vi "Select_Coreset_Idxs(CuLab).vi"(8 "error in (no error)":errorcluster, 9 "start idx":i32=-1, 10 "Sampling Ratio":sgl format="%#_13g", 11 "Features (embeddings)":refnum<class "T2D_SGL.lvclass">) -> (0 "error out":errorcluster, 2 "max distances":refnum<class "T1D_SGL.lvclass">, 3 "selected coreset idxs":i32[](array[numeric]))   [LabVIEW 2020]
uses:
  <vilib>/Ngene/CuLab - GPU Accelerated Toolkit/Toolkit/Low_Level/Tensor_Classes/T_Children/T2D/T2D_Children/T2D_SGL/T2D_SGL.lvclass
  C:/Program Files/National Instruments/LabVIEW 2020/vi.lib/Ngene/CuLab - GPU Accelerated Toolkit/Toolkit/Low_Level/Tensor_Classes/T_Children/T2D/T2D.lvclass
  <vilib>/Ngene/CuLab - GPU Accelerated Toolkit/Toolkit/Low_Level/Tensor_Classes/T_Children/T1D/T1D_Children/T1D_SGL/T1D_SGL.lvclass
  C:/Program Files/National Instruments/LabVIEW 2020/vi.lib/Ngene/CuLab - GPU Accelerated Toolkit/Toolkit/Low_Level/Tensor_Classes/T_Children/T1D/T1D.lvclass
  C:/Program Files/National Instruments/LabVIEW 2020/vi.lib/Ngene/CuLab - GPU Accelerated Toolkit/Toolkit/Low_Level/Tensor_Classes/Tensor.lvclass
  <vilib>/Ngene/CuLab - GPU Accelerated Toolkit/Toolkit/API/Array/Controls/Array_Major.ctl
  <vilib>/Ngene/CuLab - GPU Accelerated Toolkit/Toolkit/API/Array/Array Size/CU_Array_Size_T2D.vi
  <vilib>/Ngene/CuLab - GPU Accelerated Toolkit/Toolkit/API/Signal Processing/Signal Generation/Ramp Pattern/T1D/CU_Ramp_Pattern_T1D_SGL.vi
  <vilib>/Ngene/CuLab - GPU Accelerated Toolkit/Toolkit/API/Numeric/Conversion  (API)/I32/CU_To_I32_T1D.vi
  <vilib>/Ngene/CuLab - GPU Accelerated Toolkit/Toolkit/Low_Level/Tensor_Classes/T_Children/T1D/T1D_Children/T1D_I32/Pull.vi
  <vilib>/Ngene/CuLab - GPU Accelerated Toolkit/Toolkit/API/Numeric/Square/T2D/CU_Square_T2D_SGL.vi
  <vilib>/Ngene/CuLab - GPU Accelerated Toolkit/Toolkit/API/Array/Array Size/CU_Array_Size_T1D.vi
  <vilib>/Ngene/CuLab - GPU Accelerated Toolkit/Toolkit/API/Array/Index Array Subset/T2D/CU_Index_Array_Subset_T2D_SGL.vi
  <vilib>/Ngene/CuLab - GPU Accelerated Toolkit/Toolkit/API/Comparison/Max Min/T1D/CU_Max_Min_T1D_SGL.vi
  <vilib>/Ngene/CuLab - GPU Accelerated Toolkit/Toolkit/API/Array/Array Max Min/T1D/CU_Array_Max_Min_T1D_SGL.vi
  <vilib>/Ngene/CuLab - GPU Accelerated Toolkit/Toolkit/API/Array/Replace Array Element/T1D/CU_Replace_Array_Element_T1D_SGL.vi
  <vilib>/Ngene/CuLab - GPU Accelerated Toolkit/Toolkit/CuLab.lvlib
  C:/Program Files/National Instruments/LabVIEW 2020/vi.lib/Ngene/CuLab - GPU Accelerated Toolkit/Toolkit/Low_Level/Tensor_Classes/T_Children/T2D/T2D_Children/T2D_SGL/T2D_SGL.lvclass
  C:/Program Files/National Instruments/LabVIEW 2020/vi.lib/Ngene/CuLab - GPU Accelerated Toolkit/Toolkit/Low_Level/Tensor_Classes/T_Children/T1D/T1D_Children/T1D_SGL/T1D_SGL.lvclass
  <vilib>/Ngene/CuLab - GPU Accelerated Toolkit/Toolkit/Low_Level/Tensor_Classes/T_Children/T1D/T1D_Children/T1D_I32/T1D_I32.lvclass
  <vilib>/Ngene/Deep Learning Toolkit/Toolkit/Deep_Learning_Toolkit_by_Ngene.lvlib
panel:
  out "min distances":refnum<class "T1D_SGL.lvclass">
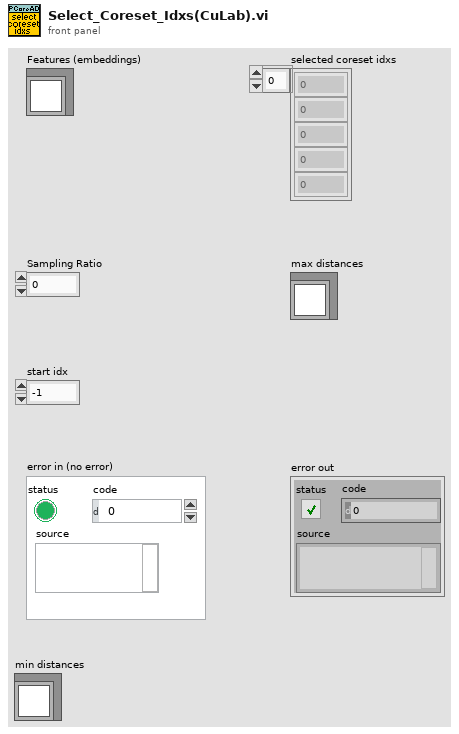
[diagram p1: front panel]
types:
  T1 = typedef "CuLab.lvlib/Array_Major.ctl" = enum16{"Row", "Column"}
  T2 = typedef "CuLab.lvlib/T2D_Dims.ctl" = cluster{"H":i32, "W":i32}
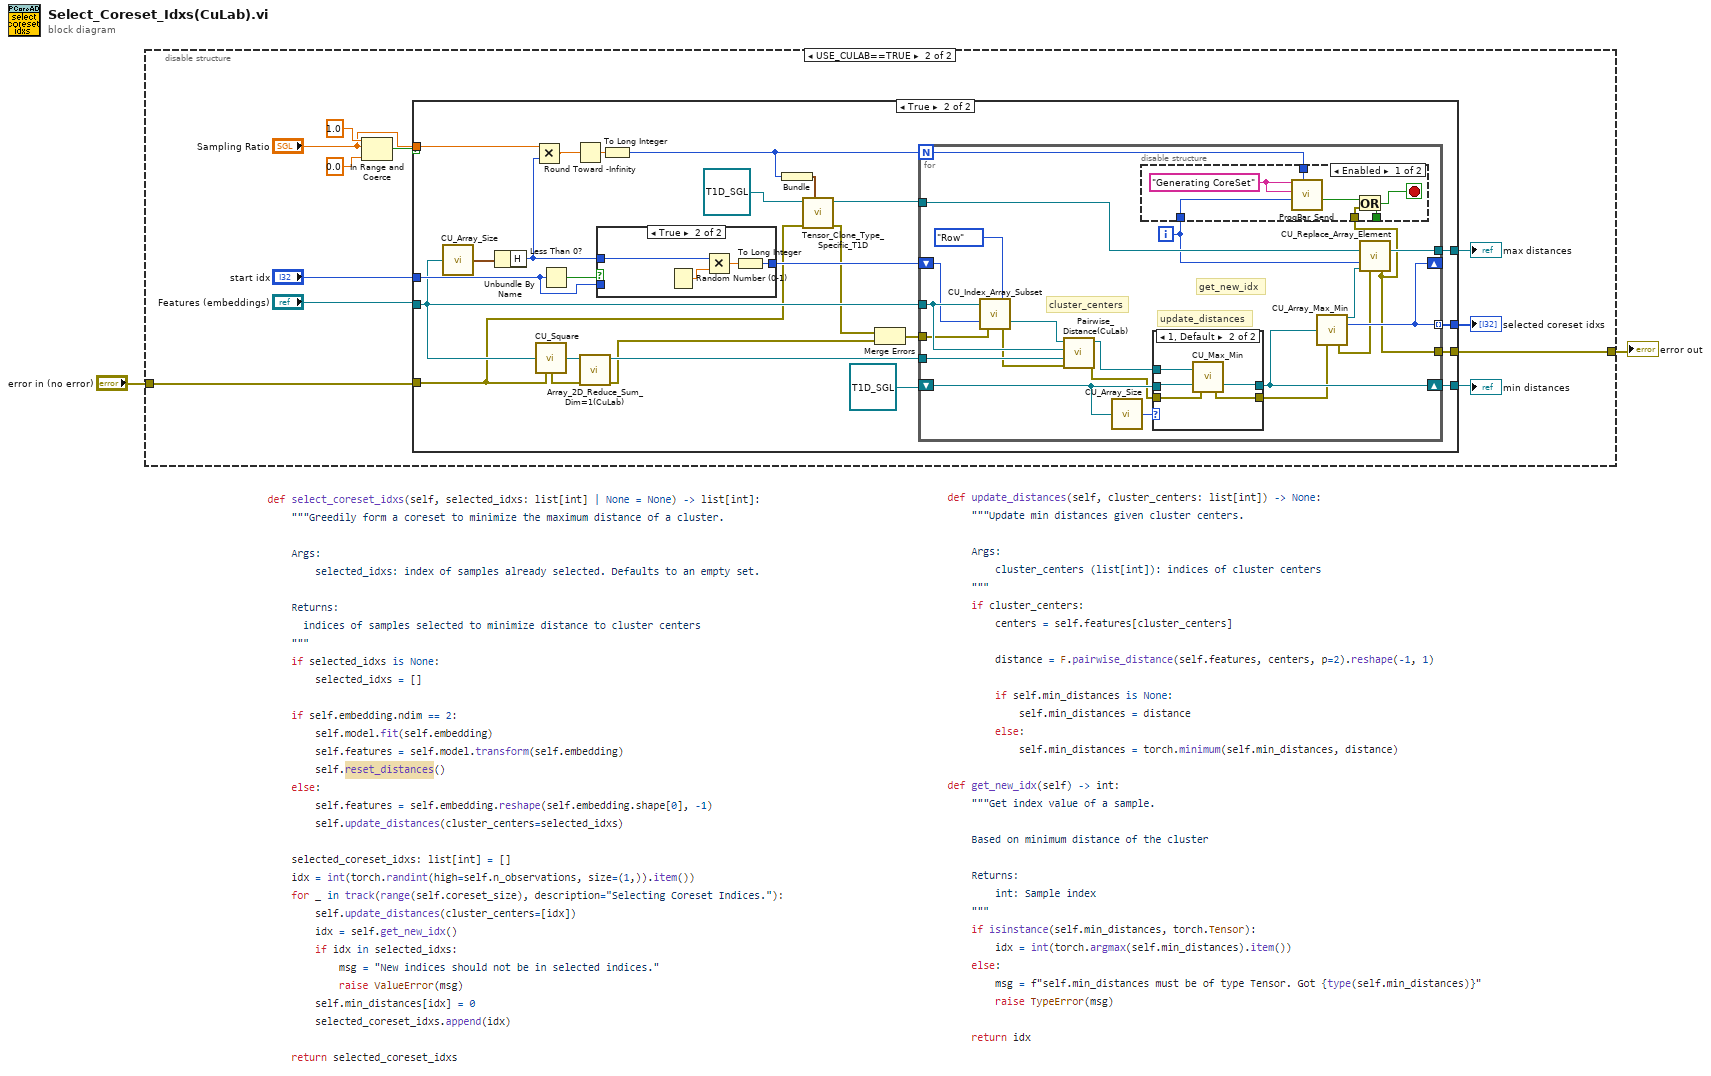
[diagram p0: block diagram]
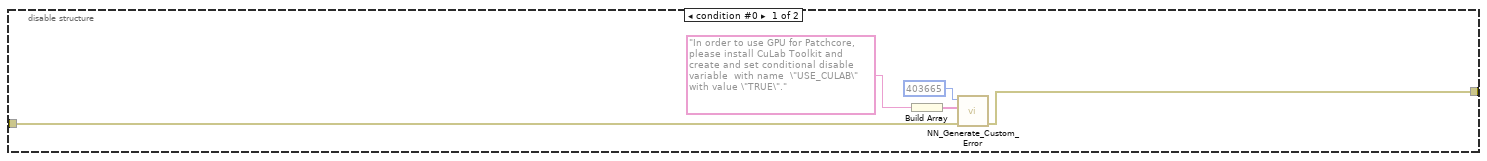
[diagram p2: hidden frame]
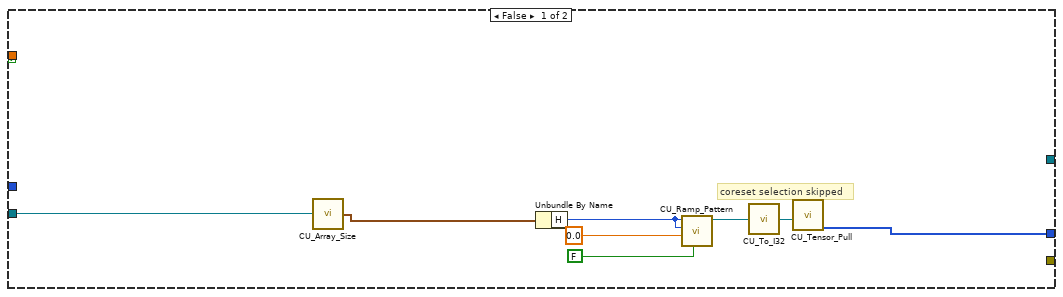
[diagram p3: hidden frame]
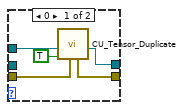
[diagram p6: hidden frame]
diagram:
  n1 = disable-structure shown="USE_CULAB==TRUE" {
    disable-tunnel: [w3 w9] -> w2
    disable-tunnel: "error in (no error)" -> [w4 w8]
    frame condition #0 {
      n2 = Build Array("In order to use GPU for Patchcore, please install CuLab Toolkit and create and set conditional disable variable  with name  \"USE_CULAB\" with value \"TRUE\"." ("Message")) -> (w6:string[])
      n3 = call <vilib>:"NN_Generate_Custom_Error.vi"("error in (no error)"=w4, "Message"=w6, "Error_code"=403665) -> ("error out"=w3:errorcluster)  [unwired: 8 in]
    }
    frame condition #1 (active) {
      n4 = In Range and Coerce(upper limit=sgl 1.0, x="Sampling Ratio", lower limit=sgl 0.0) -> (In Range?=w12:bool)  [unwired: 1 out]
      n5 = case shown="True" w12 {
        tunnel: [w20 w51] -> w18
        tunnel: [_ w50] -> w17
        tunnel: "start idx" -> [_ w47]
        tunnel: "Features (embeddings)" -> [w25 w39]
        tunnel: "Sampling Ratio" -> [_ w42]
        tunnel: [_ w33] -> w10
        tunnel: w8 -> [_ w31]
        tunnel: [_ w28] -> w9
        frame False {
          # "coreset selection skipped"
          n6 = call-poly <vilib>:"CU_Array_Size.vi"("Tensor"=w25) -> ("T2D_Dims"=w26:T2)  [unwired: 14 in]
          n7 = Unbundle By Name(w26) -> ("H"=w19:i32)
          n8 = call-poly <vilib>:"CU_Ramp_Pattern.vi"("exclude end?"=FALSE, "start"=sgl 0.0, "end"=w19, "samples"=w19) -> ("Ramp Pattern"=w22:refnum<class "T1D_SGL.lvclass">)  [unwired: 6 in, 1 out]
          n9 = call-poly <vilib>:"CU_To_I32.vi"("Tensor in"=w22) -> ("Dest out"=w21:refnum<class "T1D_I32.lvclass">)  [unwired: 13 in, 1 out]
          n10 = call-poly <vilib>:"CU_Tensor_Pull.vi"("T1D_I32 in"=w21) -> ("Dest out"=w20:i32[])  [unwired: 8 in, 2 out]
        }
        frame True {
          n11 = call-poly <vilib>:"CU_Array_Size.vi"("Tensor"=w39) -> ("T2D_Dims"=w41:T2)  [unwired: 14 in]
          n12 = Unbundle By Name(w41) -> ("H"=w40:i32)
          n13 = Multiply(x=w42, y=w40) -> (x*y=w43:sgl)
          n14 = call-poly <vilib>:"CU_Square.vi"("x"=w39, "error in (no error)"=w31) -> ("Dest out"=w46:refnum<class "T2D_SGL.lvclass">, "error out"=w32:errorcluster)  [unwired: 12 in]
          n15 = Less Than 0?(x=w47) -> (x < 0?=w48:bool)
          n16 = Round Toward -Infinity(1:w43) -> (0:w44:sgl)
          n17 = call "Array_2D_Reduce_Sum_Dim=1(CuLab).vi"("error in (no error)"=w32, "x"=w46) -> ("error out"=w27:errorcluster, "y out"=w45:refnum<class "T1D_SGL.lvclass">)  [unwired: 8 in]
          n18 = case shown="True" w48 {
            tunnel: w40 -> [_ w54]
            tunnel: [w52 w53] -> w49
            tunnel: w47 -> [w52 _]
            frame False {
            }
            frame True {
              n19 = Random Number (0-1)() -> (number: 0 to 1=w56:dbl)
              n20 = Multiply(x=w54, y=w56) -> (x*y=w55:dbl)
              n21 = To Long Integer(number=w55) -> (32bit integer=w53:i32)
            }
          }
          n22 = To Long Integer(number=w44) -> (32bit integer=w35:i32)
          n23 = Bundle(w35) -> (w37:cluster{i32})  [unwired: 1 in]
          n24 = call <vilib>:"Tensor_Clone_Type_Specific_T1D.vi"("Dest_Tensor_Dims"=w37, "error in (no error)"=w31, "Dest_Tensor"=refnum<class "T1D_SGL.lvclass"> refnum ("y out")) -> ("error out"=w30:errorcluster, "Dest_Tensor out"=w34:refnum<class "T1D_SGL.lvclass">)  [unwired: 7 in]
          n25 = Merge Errors(w30, w27) -> (w29:errorcluster)
          n26 = for {
            N: w35 -> [w72]
            tunnel: w39 -> [w71]
            shift-right: [w75] -> w50
            shift-left: refnum<class "T1D_SGL.lvclass"> refnum ("y out") -> [w78]
            shift-right: [w76] -> _
            shift-left: w49 -> [w70]
            tunnel: [w76] -> w51 mode=indexing
            tunnel: w45 -> [w74]
            tunnel: w34 -> [w67]
            tunnel: [w66] -> w33
            tunnel: w29 -> [w64]
            tunnel: [w60] -> w28
            i -> [w57]
            stop <- w61 stop-if-true
            # "get_new_idx"
            # "update_distances"
            # "cluster_centers"
            n27 = call-poly <vilib>:"CU_Index_Array_Subset.vi"("Tensor in"=w71, "Index"=w70, "error in (no error)"=w64, "Row/Column Selector"=Array_Major."Row") -> ("error out"=w63:errorcluster, "Sub Tensor"=w68:refnum<class "T1D_SGL.lvclass">)  [unwired: 14 in]
            n28 = call "Pairwise_Distance(CuLab).vi"("error in (no error)"=w63, "Features norm"=w74, "Features (embeddings)"=w71, "centers"=w68) -> ("error out"=w59:errorcluster, "y out"=w73:refnum<class "T1D_SGL.lvclass">)  [unwired: 6 in]
            n29 = call-poly <vilib>:"CU_Array_Size.vi"("Tensor"=w78) -> ("size"=w77:i32)  [unwired: 14 in]
            n30 = case shown="1, Default" w77 {
              tunnel: w73 -> [w88 w94]
              tunnel: [w87 w92] -> w75
              tunnel: w78 -> [_ w93]
              tunnel: w59 -> [w86 w91]
              tunnel: [w85 w90] -> w58
              frame 0 {
                n31 = call <vilib>:"CU_Tensor_Duplicate.vi"("error in (no error)"=w86, "Copy Data?"=TRUE, "Tensor in"=w88) -> ("Duplicate out"=w87:refnum<class "T1D_SGL.lvclass">, "error out"=w85:errorcluster)  [unwired: 7 in]
              }
              frame 1, Default {
                n32 = call-poly <vilib>:"CU_Max_Min.vi"("X"=w94, "Y"=w93, "error in (no error)"=w91) -> ("error out"=w90:errorcluster, "Min (X, Y)"=w92:refnum<class "T1D_SGL.lvclass">)  [unwired: 14 in, 1 out]
              }
            }
            n33 = call-poly <vilib>:"CU_Array_Max_Min.vi"("Tensor in"=w75, "error in (no error)"=w58) -> ("Max Dest out"=w65:refnum<class "T0D_SGL.lvclass">, "Max Index"=w76:i32, "error out"=w62:errorcluster)  [unwired: 9 in, 2 out]
            n34 = call-poly <vilib>:"CU_Replace_Array_Element.vi"("Tensor in"=w67, "Index"=w57, "New Element"=w65, "error in (no error)"=w62) -> ("Tensor out"=w66:refnum<class "T1D_SGL.lvclass">, "error out"=w60:errorcluster)  [unwired: 10 in]
            n35 = disable-structure shown="Enabled" {
              disable-tunnel: w72 -> [w84 _]
              disable-tunnel: [w82 _] -> w61
              disable-tunnel: w60 -> [w81 _]
              disable-tunnel: w57 -> [w79 _]
              frame Enabled {
                w80 = "Generating CoreSet" ("ProgBar Label")
                n36 = call "ProgBar_Send.vi"("Max Number Of Iterations"=w84, "Current Iteration"=w79, "ProgBar Label"=w80, "ProgBar Que Name"=w80) -> ("Cancelled?"=w83:bool)  [unwired: 6 in, 1 out]
                n37 = Or(x=w83, y=w81) -> (x .or. y?=w82:bool)
              }
              frame Disabled {
              }
            }
          }
        }
      }
      "selected coreset idxs" <- w18
      "min distances" <- w17
      "max distances" <- w10
    }
  }
  "error out" <- w2
